vi "reset_tilt_stage.vi"() -> ()   [LabVIEW 2016]
uses:
  C:/Users/UsphereLab/Documents/GitHub/Optlev/LabView Code/Examples/Tilt Stage/CmdLib.dll
  Examples/Tilt Stage/CmdLib.dll
panel:
  out "Array":bool[](array[boolean])
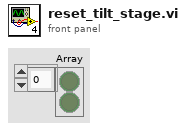
[diagram p1: front panel]
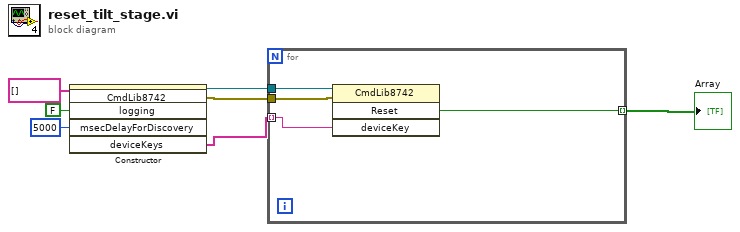
[diagram p0: block diagram]
diagram:
  n1 = constructor class="CmdLib8742"("logging"=FALSE, "msecDelayForDiscovery"=5000, "deviceKeys"=string[] []) -> (reference out=w2:refnum<k24>, error out=w1:errorcluster, "deviceKeys"=w4:string[])  [unwired: 3 in, 3 out]
  n2 = for {
    tunnel: w4 -> [w11] mode=indexing
    tunnel: [w10] -> w3 mode=indexing
    tunnel: w2 -> [w9]
    tunnel: w1 -> [w8]
    n3 = invoke class="CmdLib8742" method="Reset"(reference=w9, error in=w8, "deviceKey"=w11) -> ("Reset"=w10:bool)  [unwired: 1 in, 3 out]
  }
  "Array" <- w3
